vi "Comp_Tens Inspection.vi"(5 "Value":string[][](array[string]), 7 "분해능":string, 8 "error in (no error)":errorcluster caption="에러 입력(에러 없음)", 9 "Spec":string[][](array[string]), 10 "Condition":string[][](array[string]), 11 "STD":string[][](array[string])) -> (0 "error out":errorcluster caption="에러 출력", 1 "사용기준추":string[][](array[string]), 2 "Value out":string[][](array[string]), 3 "색상 배열":u32[][](array[numeric]))   [LabVIEW 2020]
uses:
  Controls/Cmd_File path.ctl
  Controls/Cmd_File Type.ctl
  <vilib>/Utility/file.llb/Read Delimited Spreadsheet (string).vi
  Public/Polymorph/Data Class_2D Str.vi
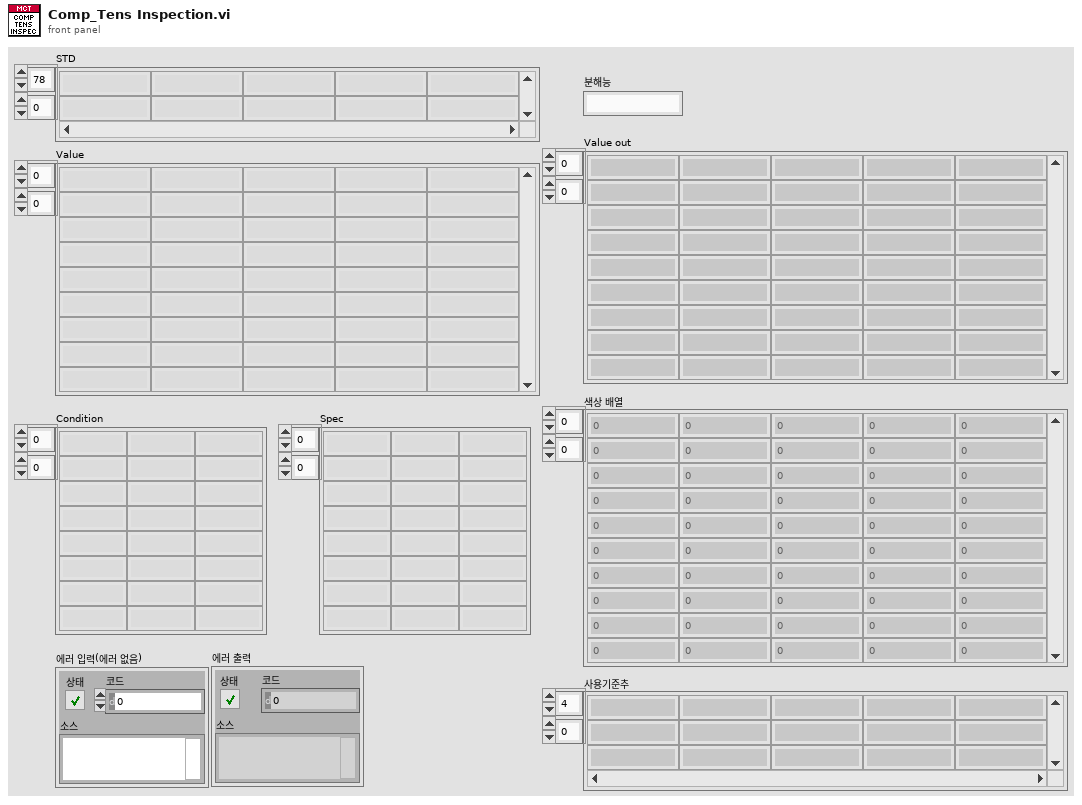
[diagram p1: front panel]
types:
  T1 = typedef "Cmd_File Type.ctl" = enum16{"엑셀", "엑셀(2003)", "텍스트", "설정", "2진", "VI", "CSV", "LOG", "폴더"}
  T2 = typedef "Cmd_File path.ctl" = enum16{"에러로그", "데이터파일경로", "성적서원본", "지난성적서", "Data Files", "경로생성", "Updater", "Template", "설정파일경로", "FTP Upload", "Update 경로", "어플리케이션"}
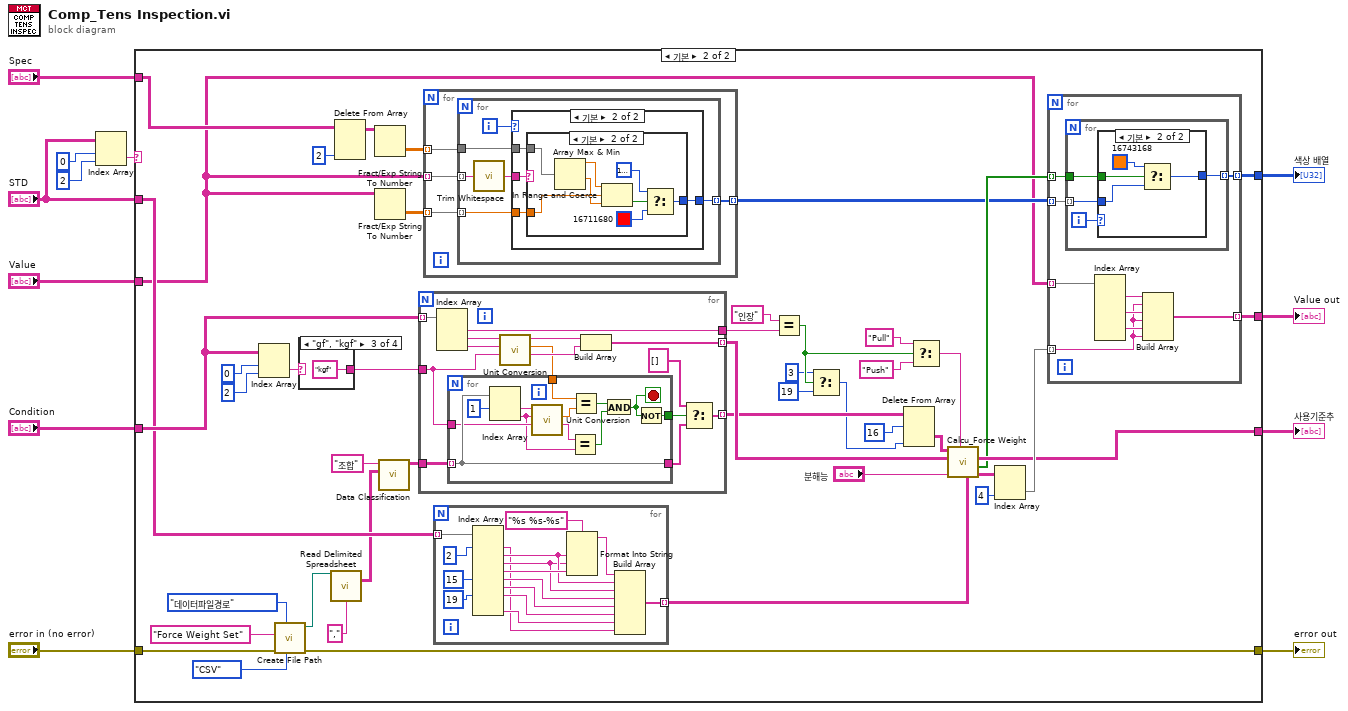
[diagram p0: block diagram]
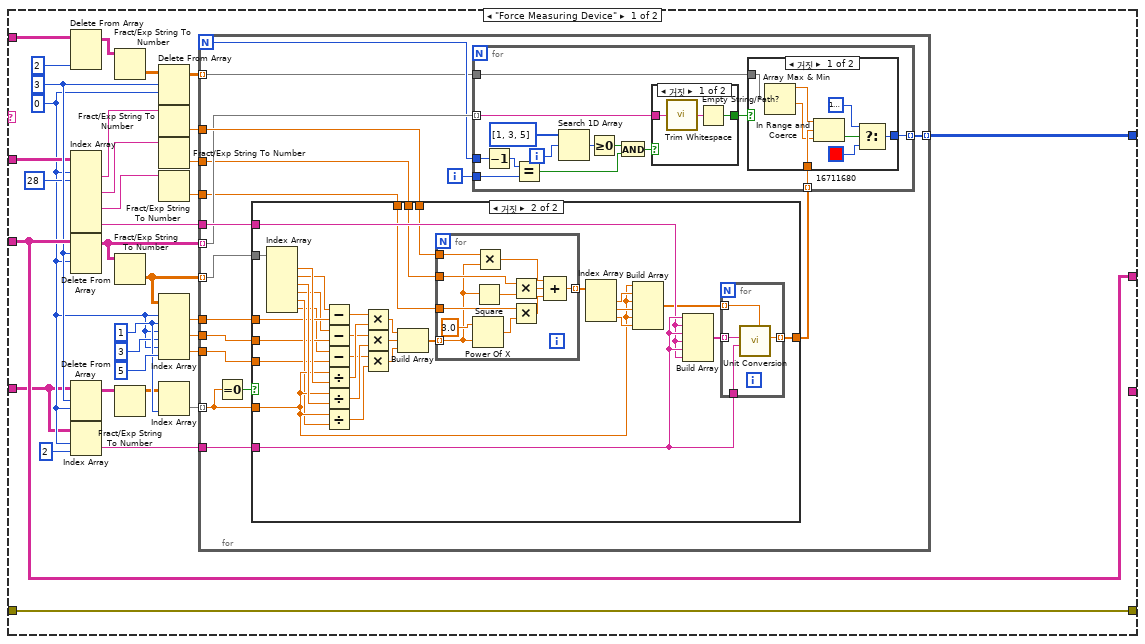
[diagram p2: hidden frame]
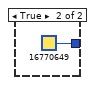
[diagram p3: hidden frame]
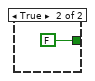
[diagram p4: hidden frame]
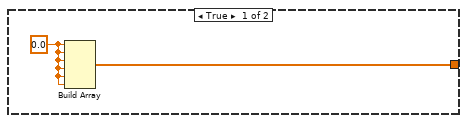
[diagram p5: hidden frame]
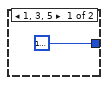
[diagram p6: hidden frame]
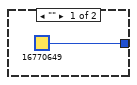
[diagram p7: hidden frame]
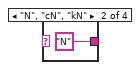
[diagram p10: hidden frame]
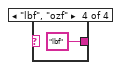
[diagram p11: hidden frame]
diagram:
  n1 = Index Array(array="STD", index (row)=0 ("비활성화된 인덱스 (행)"), index (col)=2 ("비활성화된 인덱스 (열)")) -> (element=w3:string)
  n2 = case shown="기본" w3 {
    tunnel: "STD" -> [w29 w173]
    tunnel: "Spec" -> [w19 w183]
    tunnel: "Condition" -> [w15 w174]
    tunnel: [w35 w163] -> w10
    tunnel: "Value" -> [w34 w141]
    tunnel: [w34 w166] -> w8
    tunnel: "error in (no error)" -> [w33 w159]
    tunnel: [w33 w158] -> w6
    tunnel: [_ w165] -> w1
    frame "Force Measuring Device" {
      w32 = 1 ("인덱스 (행)")
      w31 = 3 ("길이")
      w20 = 0 ("인덱스 (행)")
      n3 = Delete From Array(array=w19, index (col)=2 ("비활성화된 인덱스 (열)")) -> (array with subset deleted=w17:string[][])  [unwired: 2 in, 1 out]
      n4 = Index Array(array=w29, index (row) #1=w20, index (col) #1=28 ("비활성화된 인덱스 (열)")) -> (element #1=w27:string, element #2=w26:string, element #3=w25:string, element #4=w28:string)  [unwired: 6 in]
      n5 = Delete From Array(array=w34, length=w31, index (row)=w20) -> (array with subset deleted=w37:string[][])  [unwired: 1 in, 1 out]
      n6 = Delete From Array(array=w15, length=w31, index (row)=w20) -> (array with subset deleted=w14:string[][])  [unwired: 1 in, 1 out]
      n7 = Index Array(array=w15, index (row)=w20, index (col)=2 ("비활성화된 인덱스 (열)")) -> (element=w39:string)
      n8 = Fract/Exp String To Number(string=w17) -> (number=w16:dbl[][])  [unwired: 3 in, 1 out]
      n9 = Fract/Exp String To Number(string=w37) -> (number=w38:dbl[][])  [unwired: 3 in, 1 out]
      n10 = Fract/Exp String To Number(string=w14) -> (number=w13:dbl[][])  [unwired: 3 in, 1 out]
      n11 = Delete From Array(array=w16, length=w31, index (row)=w20) -> (array with subset deleted=w36:dbl[][])  [unwired: 1 in, 1 out]
      n12 = Fract/Exp String To Number(string=w27) -> (number=w24:dbl)  [unwired: 3 in, 1 out]
      n13 = Fract/Exp String To Number(string=w26) -> (number=w23:dbl)  [unwired: 3 in, 1 out]
      n14 = Fract/Exp String To Number(string=w25) -> (number=w22:dbl)  [unwired: 3 in, 1 out]
      n15 = Index Array(array=w38, index (row) #1=w20, index (col) #1=w32, index (row) #2=w20, index (col) #2=3 ("인덱스 (행)"), index (row) #3=w20, index (col) #3=5 ("인덱스 (행)")) -> (element #1=w41:dbl, element #2=w42:dbl, element #3=w43:dbl)
      n16 = Index Array(array=w13, index (col)=w32) -> (element=w45:dbl[])  [unwired: 1 in]
      n17 = for {
        N -> [w53]
        tunnel: w38 -> [w62] mode=indexing
        tunnel: w41 -> [w61]
        tunnel: w42 -> [w60]
        tunnel: w43 -> [w59]
        tunnel: w45 -> [w47] mode=indexing
        tunnel: w24 -> [w58]
        tunnel: w28 -> [w57]
        tunnel: w39 -> [w56]
        tunnel: w37 -> [w55] mode=indexing
        tunnel: w36 -> [w52] mode=indexing
        tunnel: [w50] -> w35 mode=indexing
        tunnel: w23 -> [w49]
        tunnel: w22 -> [w48]
        i -> [w54]
        n18 = Equal To 0?(x=w47) -> (x = 0?=w46:bool)
        n19 = case shown="거짓" w46 {
          tunnel: w62 -> [_ w124]
          tunnel: [w91 w111] -> w51
          tunnel: w61 -> [_ w102]
          tunnel: w60 -> [_ w101]
          tunnel: w59 -> [_ w100]
          tunnel: w47 -> [_ w109]
          tunnel: w58 -> [_ w94]
          tunnel: w57 -> [_ w118]
          tunnel: w56 -> [_ w119]
          tunnel: w49 -> [_ w93]
          tunnel: w48 -> [_ w92]
          frame True {
            w90 = 0.0 ("원소")
            n20 = Build Array(w90, w90, w90, w90, w90, w90) -> (w91:dbl[])
          }
          frame False {
            n21 = Index Array(array=w124) -> (element #1=w117:dbl, element #2=w103:dbl, element #3=w110:dbl, element #4=w99:dbl, element #5=w108:dbl, element #6=w98:dbl)  [unwired: 6 in]
            n22 = Subtract(x=w103, y=w102) -> (x-y=w97:dbl)
            n23 = Subtract(x=w99, y=w101) -> (x-y=w96:dbl)
            n24 = Subtract(x=w98, y=w100) -> (x-y=w95:dbl)
            n25 = Divide(x=w109, y=w117) -> (x/y=w116:dbl)
            n26 = Divide(x=w109, y=w110) -> (x/y=w107:dbl)
            n27 = Divide(x=w109, y=w108) -> (x/y=w106:dbl)
            n28 = Multiply(x=w97, y=w116) -> (x*y=w115:dbl)
            n29 = Multiply(x=w96, y=w107) -> (x*y=w105:dbl)
            n30 = Multiply(x=w95, y=w106) -> (x*y=w104:dbl)
            n31 = Build Array(w115, w105, w104) -> (w113:dbl[])
            n32 = for {
              tunnel: w94 -> [w139]
              tunnel: w93 -> [w138]
              tunnel: w92 -> [w136]
              tunnel: w113 -> [w129] mode=indexing
              tunnel: [w130] -> w112 mode=indexing
              n33 = Power Of X(1:w129, 2:3.0 ("y")) -> (0:w134:dbl)
              n34 = Square(x=w129) -> (x^2=w137:dbl)
              n35 = Multiply(x=w139, y=w129) -> (x*y=w133:dbl)
              n36 = Multiply(x=w138, y=w137) -> (x*y=w132:dbl)
              n37 = Multiply(x=w136, y=w134) -> (x*y=w131:dbl)
              n38 = Compound Arithmetic op=ADD(w133, w132, w131) -> (w130:dbl)
            }
            n39 = Index Array(array=w112) -> (element #1=w123:dbl, element #2=w122:dbl, element #3=w121:dbl)  [unwired: 3 in]
            n40 = Build Array(w109, w123, w109, w122, w109, w121) -> (w114:dbl[])
            n41 = Build Array(w119, w118, w119, w118, w119, w118) -> (w120:string[])
            n42 = for {
              tunnel: w114 -> [w128] mode=indexing
              tunnel: w119 -> [w127]
              tunnel: [w126] -> w111 mode=indexing
              tunnel: w120 -> [w125] mode=indexing
              n43 = call "Unit Conversion.vi"("입력값 (옵션)"=w128, "환산단위"=w127, "입력단위"=w125) -> ("환산값 (DBL)"=w126:dbl)  [unwired: 3 in, 5 out]
            }
          }
        }
        n44 = for {
          tunnel: w55 -> [w63] mode=indexing
          tunnel: w53 -> [w75]
          tunnel: w54 -> [w74]
          tunnel: w52 -> [w64]
          tunnel: w51 -> [w66] mode=indexing
          tunnel: [w65] -> w50 mode=indexing
          i -> [w73]
          n45 = Decrement(x=w75) -> (x-1=w76:i32)
          n46 = Equal?(x=w76, y=w74) -> (x = y?=w69:bool)
          n47 = Search 1D Array(1D array=i32[] [1, 3, 5], element=w73) -> (index of element=w71:i32)  [unwired: 1 in]
          n48 = Greater Or Equal To 0?(x=w71) -> (x >= 0?=w70:bool)
          n49 = And(x=w70, y=w69) -> (x .and. y?=w68:bool)
          n50 = case shown="거짓" w68 {
            tunnel: [w87 FALSE] -> w67
            tunnel: w63 -> [w88 _]
            frame False {
              n51 = call <vilib>:"Trim Whitespace.vi"("string"=w88) -> ("trimmed string"=w86:string)  [unwired: 1 in]
              n52 = Empty String/Path?(string/path=w86) -> (empty?=w87:bool)
            }
            frame True {
            }
          }
          n53 = case shown="거짓" w67 {
            tunnel: w66 -> [w84 _]
            tunnel: [w81 u32 16770649] -> w65
            tunnel: w64 -> [w79 _]
            frame False {
              n54 = Array Max & Min(array=w79) -> (max value=w78:dbl, min value=w77:dbl)  [unwired: 2 out]
              n55 = In Range and Coerce(upper limit=w78, x=w84, lower limit=w77) -> (In Range?=w83:bool)  [unwired: 1 out]
              n56 = Select(t=u32 16777226, s=w83, f=u32 16711680) -> (s? t:f=w81:u32)
            }
            frame True {
            }
          }
        }
      }
    }
    frame Default {
      n57 = Index Array(array=w174, index (row)=0 ("인덱스 (행)"), index (col)=2 ("비활성화된 인덱스 (열)")) -> (element=w177:string)
      n58 = call "Create File Path.vi"("파일타입"=Cmd_File_Type."CSV", "항목"=Cmd_File_path."데이터파일경로", "에러 입력"=w159, "문자열 in"="Force Weight Set") -> ("error out"=w158:errorcluster, "파일경로"=w157:path)  [unwired: 4 in, 2 out]
      n59 = case shown="\"gf\", \"kgf\"" w177 {
        tunnel: [_ "N" "kgf" "lbf"] -> w176
        frame Default {
        }
        frame "N", "cN", "kN" {
        }
        frame "gf", "kgf" {
        }
        frame "lbf", "ozf" {
        }
      }
      n60 = call-poly <vilib>:"Read Delimited Spreadsheet.vi"("file path (dialog if empty)"=w157, "delimiter (\\t)"="," ("delimiter (\\t)")) -> ("all rows"=w156:string[][])  [unwired: 8 in, 5 out]
      n61 = Delete From Array(array=w183, index (col)=2 ("비활성화된 인덱스 (열)")) -> (array with subset deleted=w170:string[][])  [unwired: 2 in, 1 out]
      n62 = Fract/Exp String To Number(string=w170) -> (number=w140:dbl[][])  [unwired: 3 in, 1 out]
      n63 = Fract/Exp String To Number(string=w141) -> (number=w142:dbl[][])  [unwired: 3 in, 1 out]
      n64 = call-poly "Data Classification.vi"("DATA 입력"=w156, "검색 문자열"="조합") -> ("DATA 출력"=w180:string[][])  [unwired: 5 in, 4 out]
      n65 = for {
        tunnel: w180 -> [w258]
        tunnel: w176 -> [w256]
        tunnel: w174 -> [w257] mode=indexing
        tunnel: [w248] -> w152 mode=indexing
        tunnel: [w250] -> w171 mode=indexing
        tunnel: [w249] -> w148
        n66 = Index Array(array=w257) -> (element #1=w249:string, element #2=w247:string, element #3=w252:string)  [unwired: 3 in]
        n67 = call "Unit Conversion.vi"("환산단위"=w256, "입력단위"=w252, "입력값"=w247) -> ("환산단위"=w251:string, "환산값 (DBL)"=w245:dbl, "환산값 (string)"=w246:string)  [unwired: 3 in, 3 out]
        n68 = for {
          tunnel: [w270] -> w255
          tunnel: w258 -> [w269] mode=indexing
          tunnel: [w269] -> w253
          tunnel: w256 -> [w266]
          tunnel: w245 -> [w259]
          stop <- w261 stop-if-true
          n69 = Index Array(array=w269, index #1=1 ("인덱스")) -> (element #1=w267:string, element #2=w264:string)  [unwired: 1 in]
          n70 = call "Unit Conversion.vi"("환산단위"=w266, "입력단위"=w264, "입력값"=w267) -> ("환산단위"=w265:string, "환산값 (DBL)"=w260:dbl)  [unwired: 3 in, 4 out]
          n71 = Equal?(x=w265, y=w264) -> (x = y?=w262:bool)
          n72 = Equal?(x=w259, y=w260) -> (x = y?=w263:bool)
          n73 = And(x=w263, y=w262) -> (x .and. y?=w261:bool)
          n74 = Not(x=w261) -> (.not. x?=w270:bool)
        }
        n75 = Build Array(w246, w251) -> (w250:string[])
        n76 = Select(t=string[] [] ("f"), s=w255, f=w253) -> (s? t:f=w248:string[])
      }
      n77 = for {
        tunnel: [w188] -> w143 mode=indexing
        tunnel: w142 -> [w187] mode=indexing
        tunnel: w141 -> [w186] mode=indexing
        tunnel: w140 -> [w185] mode=indexing
        n78 = for {
          tunnel: w186 -> [w191] mode=indexing
          tunnel: w185 -> [w194]
          tunnel: [w193] -> w188 mode=indexing
          tunnel: w187 -> [w192] mode=indexing
          i -> [w189]
          n79 = call <vilib>:"Trim Whitespace.vi"("string"=w191) -> ("trimmed string"=w190:string)  [unwired: 1 in]
          n80 = case shown="기본" w189 {
            tunnel: w194 -> [_ w199]
            tunnel: [u32 16777226 w198] -> w193
            tunnel: w192 -> [_ w197]
            tunnel: w190 -> [_ w196]
            frame 1, 3, 5 {
            }
            frame Default {
              n81 = case shown="기본" w196 {
                tunnel: w199 -> [_ w208]
                tunnel: [u32 16770649 w207] -> w198
                tunnel: w197 -> [_ w206]
                frame "" {
                }
                frame Default {
                  n82 = Array Max & Min(array=w208) -> (max value=w202:dbl, min value=w201:dbl)  [unwired: 2 out]
                  n83 = In Range and Coerce(upper limit=w202, x=w206, lower limit=w201) -> (In Range?=w205:bool)  [unwired: 1 out]
                  n84 = Select(t=u32 16777226, s=w205, f=u32 16711680) -> (s? t:f=w207:u32)
                }
              }
            }
          }
        }
      }
      n85 = for {
        tunnel: w173 -> [w238] mode=indexing
        tunnel: [w237] -> w172 mode=indexing
        n86 = Index Array(array=w238, index #1=2 ("인덱스"), index #5=15 ("인덱스"), index #7=19 ("인덱스")) -> (element #1=w227:string, element #2=w230:string, element #3=w229:string, element #4=w241:string, element #5=w235:string, element #6=w234:string, element #7=w232:string, element #9=w231:string)  [unwired: 6 in, 1 out]
        n87 = Format Into String(format string="%s %s-%s" ("포맷 문자열"), w230, w229, w241) -> (resulting string=w239:string)  [unwired: 2 in, 1 out]
        n88 = Build Array(w239, w230, w229, w235, w234, w232, w231, w227) -> (w237:string[])
      }
      n89 = Equal?(x="인장" ("y"), y=w148) -> (x = y?=w147:bool)
      n90 = Select(t=3 ("비활성화된 인덱스 (열)"), s=w147, f=19 ("비활성화된 인덱스 (열)")) -> (s? t:f=w146:i32)
      n91 = Delete From Array(array=w152, length=16 ("길이"), index (col)=w146) -> (deleted portion=w150:string[][])  [unwired: 1 in, 1 out]
      n92 = Select(t="Pull" ("방향"), s=w147, f="Push" ("방향")) -> (s? t:f=w154:string)
      n93 = call "Calcu_Force Weight.vi"("기준기 데이터"=w172, "방향"=w154, "분해능"="분해능", "Condition"=w171, "분동조합"=w150) -> ("Condition Out"=w169:string[][], "에러 배열"=w164:bool[], "사용기준추"=w165:string[][])  [unwired: 3 in, 1 out]
      n94 = Index Array(array=w169, index (col)=4 ("비활성화된 인덱스 (열)")) -> (element=w167:string[])  [unwired: 1 in]
      n95 = for {
        tunnel: w141 -> [w217] mode=indexing
        tunnel: w167 -> [w213] mode=indexing
        tunnel: [w212] -> w166 mode=indexing
        tunnel: w143 -> [w211] mode=indexing
        tunnel: w164 -> [w209] mode=indexing
        tunnel: [w210] -> w163 mode=indexing
        n96 = for {
          tunnel: w211 -> [w220] mode=indexing
          tunnel: [w219] -> w210 mode=indexing
          tunnel: w209 -> [w218]
          i -> [w221]
          n97 = case shown="기본" w221 {
            tunnel: w220 -> [w222 w225]
            tunnel: [w222 w224] -> w219
            tunnel: w218 -> [_ w226]
            frame 0, 2, 4 {
            }
            frame Default {
              n98 = Select(t=u32 16743168, s=w226, f=w225) -> (s? t:f=w224:u32)
            }
          }
        }
        n99 = Index Array(array=w217) -> (element #1=w216:string, element #3=w215:string, element #5=w214:string)  [unwired: 6 in, 3 out]
        n100 = Build Array(w216, w213, w215, w213, w214, w213) -> (w212:string[])
      }
    }
  }
  "색상 배열" <- w10
  "Value out" <- w8
  "error out" <- w6
  "사용기준추" <- w1
